vi "Drive_Utils_ConvertSpeed.vi"(2 "error in":errorcluster, 3 "Speed (m/s)":dbl) -> (0 "error out":errorcluster, 1 "Speed (-1..1)":dbl)   [LabVIEW 2009, in "Drive.lvlib" / "Drive_Utils.lvlib"]
uses:
  Drive_Utils.lvlib
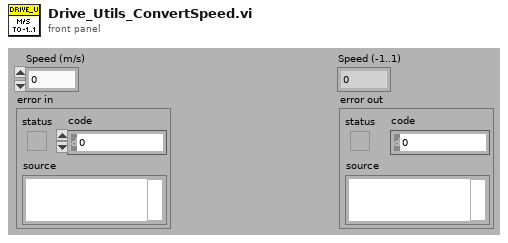
[diagram p1: front panel]
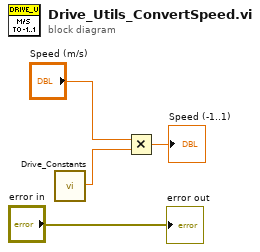
[diagram p0: block diagram]
diagram:
  n1 = call "Drive_Constants.vi"() -> ("Speed convert constant"=w4:dbl)  [unwired: 23 in, 4 out]
  n2 = Multiply(x="Speed (m/s)", y=w4) -> (x*y=→"Speed (-1..1)":dbl)
  "error out" <- "error in"
